vi "Write Data to Cell.vi"   [LabVIEW 2015]
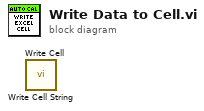
[diagram p0: block diagram]
diagram:
  n1 = call "Write Cell String.vi"() -> ()  [unwired: 10 in, 2 out]
  n2 = call "Write Cell.vi"() -> ()  [unwired: 10 in, 2 out]
